vi "Receive Transfer Data.vi"(8 "error in":errorcluster, 9 "transfer id":i32, 10 "transfer group id":i32, 11 "RDMA Transceiver in":refnum<class "RDMA Transceiver.lvclass">) -> (0 "error out":errorcluster, 1 "transfer data":u8[](array[numeric]), 3 "RDMA Transceiver out":refnum<class "RDMA Transceiver.lvclass">, 4 "valid":bool)   [LabVIEW 2020, in "RDMA.lvlib" / "RDMA Transceiver.lvclass"]
doc: "Fetches transfer data from RDMA buffer"
uses:
  RDMA Transceiver.lvclass
  <vilib>/Utility/error.llb/Clear Errors.vi
  RDMA Transceiver.lvclass/RDMA Transceiver.ctl
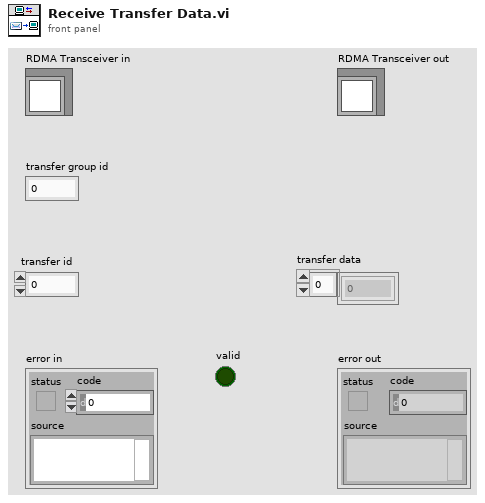
[diagram p1: front panel]
types:
  T1 = typedef "RDMA.lvlib/RDMA Transceiver.lvclass/Transfer Group Parameters.ctl" = cluster{"transfers":T2[]}
  T2 = typedef "RDMA.lvlib/RDMA Transceiver.lvclass/Transfer Parameters.ctl" = cluster{"connected session":refnum<k21>, "listener session":refnum<k21>}
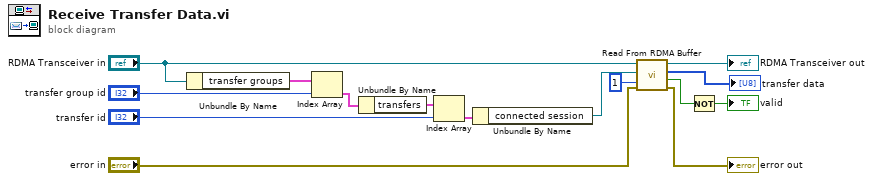
[diagram p0: block diagram]
diagram:
  n1 = Unbundle By Name("RDMA Transceiver in") -> ("transfer groups"=w15:T1[])
  n2 = Index Array(array=w15, index="transfer group id") -> (element=w13:T1)
  n3 = Unbundle By Name(w13) -> ("transfers"=w11:T2[])
  n4 = Index Array(array=w11, index="transfer id") -> (element=w10:T2)
  n5 = Unbundle By Name(w10) -> ("connected session"=w4:refnum<k21>)
  n6 = call "Read From RDMA Buffer.vi"("error in"="error in", "timeout ms (25000)"=1, "rdma session"=w4, "RDMA Transceiver in"="RDMA Transceiver in") -> ("error out"=→"error out":errorcluster, "timed out?"=w6:bool, "data"=→"transfer data":u8[], "RDMA Transceiver out"=→"RDMA Transceiver out":refnum<class "RDMA Transceiver.lvclass">)  [unwired: 4 in]
  n7 = Not(x=w6) -> (.not. x?=→"valid":bool)
